vi "Scalar FPGA Personality.vi"() -> ()   [LabVIEW 2018]
uses:
  cRIO RT/TypeDefs/Simple cluster.ctl
  cRIO RT/TypeDefs/Complex cluster.ctl
  <vilib>/rvi/Emulation/niFpgaGetClockAttributes.vi
  <vilib>/rvi/Emulation/niFpgaSctlEmulationGetInTimedLoop.vi
  <vilib>/rvi/Emulation/niFpgaEmulationReportErrorSimple.vi
  <vilib>/rvi/Emulation/niFpgaCriticalErrorInLSC.vi
panel:
  out "Complex cluster out":T1
  in  "Complex cluster in":T1
  out "Simple cluster out":T2
  in  "Simple cluster in":T2
  in  "Numeric FXP 32/16 in":fxp<+/-,32,16>
  in  "Numeric U8 in":u8
  in  "Numeric U16 in":u16
  in  "Numeric U32 in":u32
  in  "Numeric U64 in":u64
  in  "Numeric I8 in":i8
  in  "Numeric I32 in":i32
  in  "Numeric I64 in":i64
  in  "Numeric SGL in":sgl
  in  "Numeric I16 in":i16
  out "Boolean out":bool
  out "Numeric U8 out":u8
  out "Numeric U16 out":u16
  out "Numeric U32 out":u32
  out "Numeric U64 out":u64
  out "Numeric I8 out":i8
  out "Numeric I32 out":i32
  out "Numeric I64 out":i64
  out "Numeric FXP 32/16 out":fxp<+/-,32,16>
  out "Numeric SGL out":sgl
  out "Numeric I16 out":i16
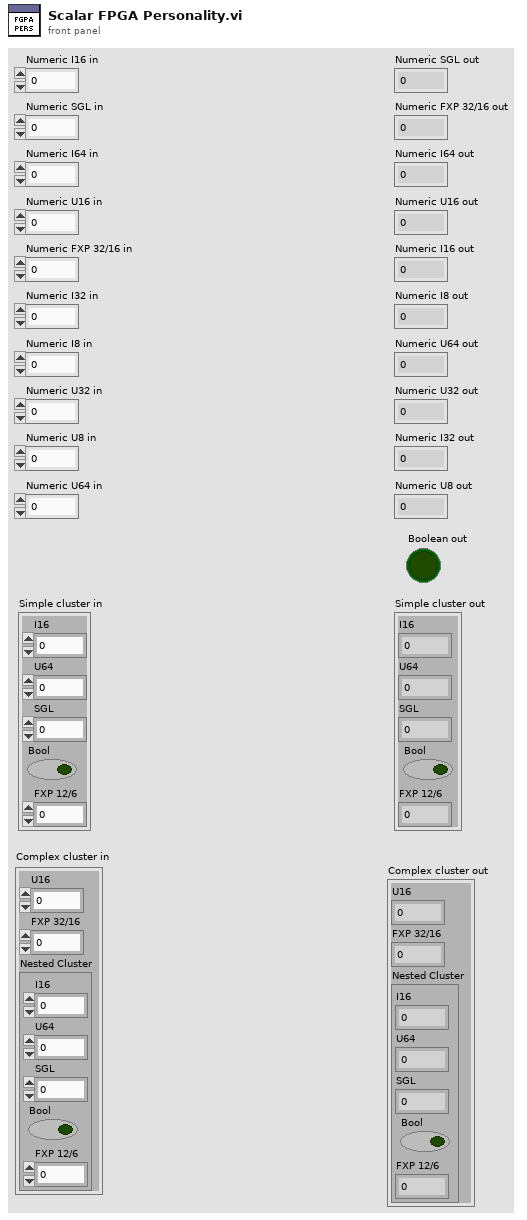
[diagram p1: front panel]
types:
  T1 = typedef "Complex cluster.ctl" = cluster{"U16":u16, "FXP 32/16":fxp<+/-,32,16>, "Nested Cluster":T2}
  T2 = typedef "Simple cluster.ctl" = cluster{"I16":i16, "U64":u64, "SGL":sgl, "Bool":bool, "FXP 12/6":fxp<+/-,12,6>}
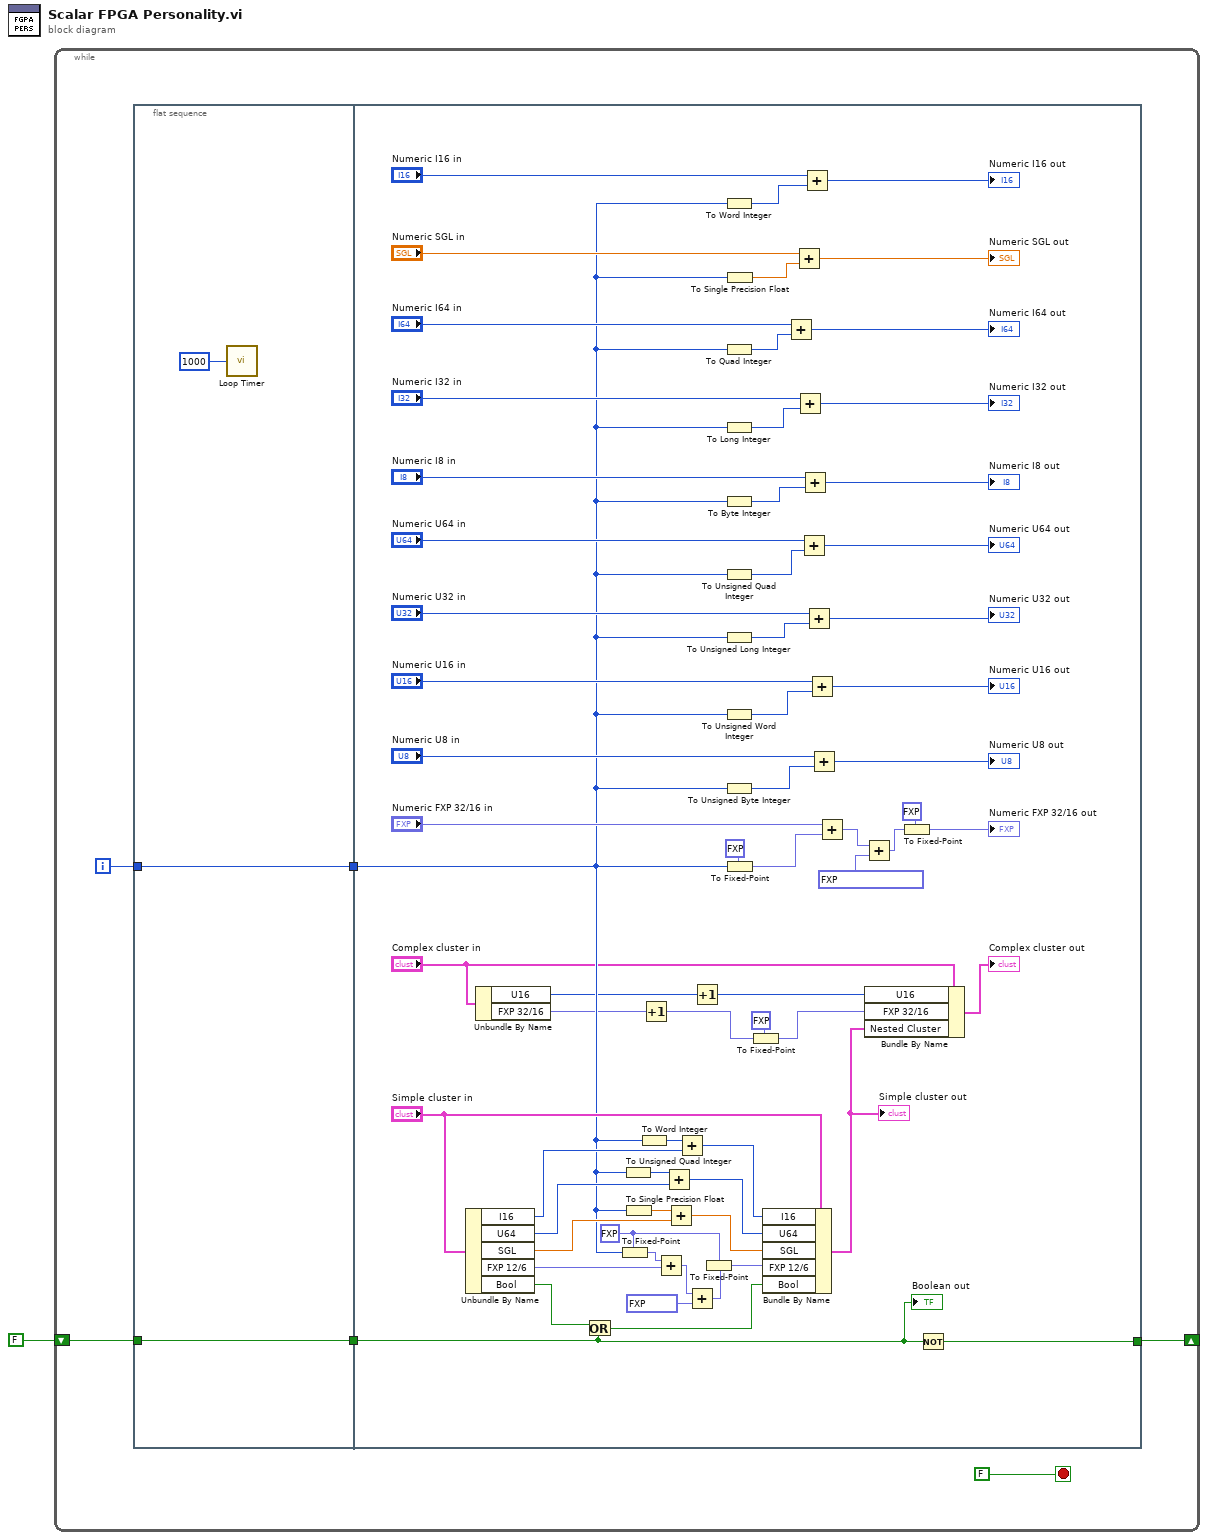
[diagram p0: block diagram]
diagram:
  n1 = while {
    shift-right: [w2] -> _
    shift-left: FALSE -> [w4]
    i -> [w6]
    stop <- FALSE stop-if-true
    n2 = flat-sequence {
      tunnel: w6 -> [w9]
      tunnel: [w9] -> w5
      tunnel: w4 -> [w8]
      tunnel: [w8] -> w3
      tunnel: w5 -> [w34]
      tunnel: w3 -> [w32]
      tunnel: [w75] -> w2
      frame #0 {
        n3 = call "Loop Timer"("Count(mSec)"=u32 1000) -> ()  [unwired: 1 out]
      }
      frame #1 {
        w15 = fxp<+/-,12,6> 0.0 ("FXP 12/6")
        n4 = Unbundle By Name("Simple cluster in") -> ("I16"=w43:i16, "U64"=w42:u64, "SGL"=w38:sgl, "FXP 12/6"=w35:fxp<+/-,12,6>, "Bool"=w31:bool)
        n5 = Unbundle By Name("Complex cluster in") -> ("U16"=w26:u16, "FXP 32/16"=w24:fxp<+/-,32,16>)
        n6 = Or(x=w31, y=w32) -> (x .or. y?=w30:bool)
        n7 = To Fixed-Point(fixed-point type=w15, number=w34) -> (fixed-point=w33:fxp<+/-,12,6>)
        n8 = To Unsigned Quad Integer(1:w34) -> (0:w41:u64)
        n9 = To Single Precision Float(number=w34) -> (single precision float=w37:sgl)
        n10 = To Word Integer(number=w34) -> (16bit integer=w44:i16)
        n11 = Increment(x=w24) -> (x+1=w17:fxp<+/-,33,17>)
        n12 = Add(x=w33, y=w35) -> (x+y=w13:fxp<+/-,13,7>)
        n13 = Add(x=w41, y=w42) -> (x+y=w39:u64)
        n14 = Add(x=w37, y=w38) -> (x+y=w36:sgl)
        n15 = Add(x=w44, y=w43) -> (x+y=w40:i16)
        n16 = Add(x=w13, y=fxp<+/-,12,6> 0.109375 ("FXP 12/6")) -> (x+y=w12:fxp<+/-,14,8>)
        n17 = Increment(x=w26) -> (x+1=w25:u16)
        n18 = To Fixed-Point(fixed-point type=w15, number=w12) -> (fixed-point=w14:fxp<+/-,12,6>)
        n19 = To Word Integer(number=w34) -> (16bit integer=w74:i16)
        n20 = To Quad Integer(1:w34) -> (0:w68:i64)
        n21 = To Long Integer(number=w34) -> (32bit integer=w65:i32)
        n22 = To Byte Integer(number=w34) -> (8bit integer=w62:i8)
        n23 = To Unsigned Quad Integer(1:w34) -> (0:w59:u64)
        n24 = To Unsigned Long Integer(number=w34) -> (unsigned 32bit integer=w56:u32)
        n25 = To Unsigned Word Integer(number=w34) -> (unsigned 16bit integer=w53:u16)
        n26 = To Unsigned Byte Integer(number=w34) -> (unsigned 8bit integer=w50:u8)
        n27 = To Single Precision Float(number=w34) -> (single precision float=w71:sgl)
        n28 = To Fixed-Point(fixed-point type=fxp<+/-,32,16> 0.0, number=w34) -> (fixed-point=w47:fxp<+/-,32,16>)
        n29 = To Fixed-Point(fixed-point type=fxp<+/-,32,16> 0.0, number=w17) -> (fixed-point=w16:fxp<+/-,32,16>)
        n30 = Bundle By Name(cluster="Simple cluster in", "I16"=w40, "U64"=w39, "SGL"=w36, "FXP 12/6"=w14, "Bool"=w30) -> (w29:T2)
        "Simple cluster out" <- w29
        n31 = Add(x="Numeric I64 in", y=w68) -> (x+y=→"Numeric I64 out":i64)
        n32 = Add(x="Numeric SGL in", y=w71) -> (x+y=→"Numeric SGL out":sgl)
        n33 = Add(x="Numeric I32 in", y=w65) -> (x+y=→"Numeric I32 out":i32)
        n34 = Add(x="Numeric U64 in", y=w59) -> (x+y=→"Numeric U64 out":u64)
        n35 = Add(x="Numeric I8 in", y=w62) -> (x+y=→"Numeric I8 out":i8)
        n36 = Add(x="Numeric I16 in", y=w74) -> (x+y=→"Numeric I16 out":i16)
        n37 = Add(x="Numeric U32 in", y=w56) -> (x+y=→"Numeric U32 out":u32)
        n38 = Add(x="Numeric U16 in", y=w53) -> (x+y=→"Numeric U16 out":u16)
        n39 = Add(x="Numeric U8 in", y=w50) -> (x+y=→"Numeric U8 out":u8)
        n40 = Add(x="Numeric FXP 32/16 in", y=w47) -> (x+y=w21:fxp<+/-,33,17>)
        n41 = Add(x=w21, y=fxp<+/-,33,17> 0.111114501953125) -> (x+y=w20:fxp<+/-,34,18>)
        n42 = Bundle By Name(cluster="Complex cluster in", "U16"=w25, "FXP 32/16"=w16, "Nested Cluster"=w29) -> (→"Complex cluster out":T1)
        n43 = To Fixed-Point(fixed-point type=fxp<+/-,32,16> 0.0, number=w20) -> (fixed-point=→"Numeric FXP 32/16 out":fxp<+/-,32,16>)
        n44 = Not(x=w32) -> (.not. x?=w75:bool)
        "Boolean out" <- w32
      }
    }
  }
